vi "UDP Data Link - Configuration Utilities - Remove System Mapping.vi"(8 "error in (no error)":errorcluster, 10 "Channel Path Destination":string, 11 "Item Ref in":T1 format="%.0x") -> (0 "error out":errorcluster, 3 "Item Ref out":T1 format="%.0x")   [LabVIEW 2015, in "UDP-Custom-Device System Explorer.lvlib"]
uses:
  UDP-Custom-Device System Explorer.lvlib
  <vilib>/NI Veristand/Custom Device API/Custom Device Item Ref.ctl
  NationalInstruments.VeriStand.SystemDefinitionAPI
  <vilib>/NI VeriStand/Custom Device API/Custom Device API.lvlib
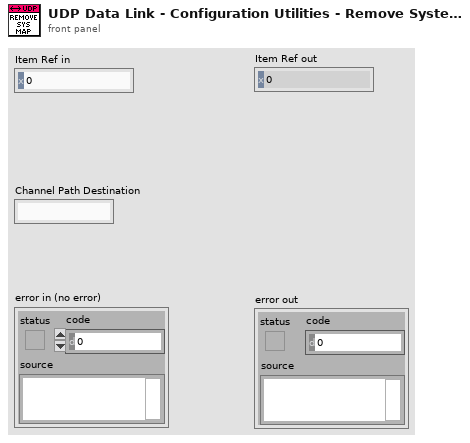
[diagram p1: front panel]
types:
  T1 = typedef "Custom Device API.lvlib/Custom Device Item Ref.ctl" = u64
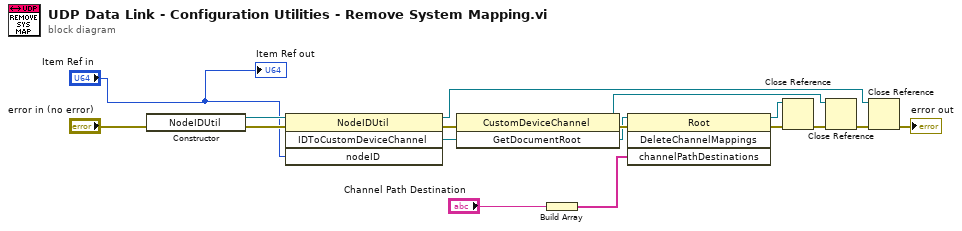
[diagram p0: block diagram]
diagram:
  n1 = constructor class="NodeIDUtil"(error in="error in (no error)") -> (reference out=w7:refnum<k24>, error out=w3:errorcluster)  [unwired: 2 in, 1 out]
  n2 = invoke class="NodeIDUtil" method="IDToCustomDeviceChannel"(reference=w7, error in=w3, "nodeID"="Item Ref in") -> (reference out=w17:refnum<k24>, error out=w10:errorcluster, "IDToCustomDeviceChannel"=w8:refnum<k24>)  [unwired: 1 in, 1 out]
  n3 = invoke class="CustomDeviceChannel" method="GetDocumentRoot"(reference=w8, error in=w10) -> (reference out=w15:refnum<k24>, error out=w11:errorcluster, "GetDocumentRoot"=w9:refnum<k24>)  [unwired: 1 in]
  n4 = Build Array("Channel Path Destination") -> (w5:string[])
  n5 = invoke class="Root" method="DeleteChannelMappings"(reference=w9, error in=w11, "channelPathDestinations"=w5) -> (reference out=w13:refnum<k24>, error out=w12:errorcluster)  [unwired: 1 in, 2 out]
  n6 = Close Reference(reference=w13, error in (no error)=w12) -> (error out=w14:errorcluster)
  n7 = Close Reference(reference=w15, error in (no error)=w14) -> (error out=w16:errorcluster)
  n8 = Close Reference(reference=w17, error in (no error)=w16) -> (error out=→"error out":errorcluster)
  "Item Ref out" <- "Item Ref in"
